vi "Analyze.vi"(8 "error in (no error)":errorcluster, 10 "Image in":T1, 11 "Analyze Total Counts in":refnum<class "Analyze Total Counts.lvclass">) -> (0 "error out":errorcluster, 1 "Result":refnum<class "Analyze Results Base.lvclass">, 2 "Image out":T1, 3 "Analyze Total Counts out":refnum<class "Analyze Total Counts.lvclass">)   [LabVIEW 2020, in "Analyze.lvlib" / "Analyze Total Counts.lvclass"]
uses:
  Analyze Total Counts.lvclass
  C:/POLARIS Programme/POLARIS-AS-3-Cams/Submodules/HIJ Vision/Analyze/Analyze Classes/Analyze BaseClass/Analyze BaseClass/Analyze BaseClass.lvclass
  <vilib>/vision/Image Controls.llb/IMAQ Image.ctl
  Results and Overlays/Results Base/Analyze Results Base.lvclass
  Results and Overlays/Results Total Counts/Analyze Results Total Counts.lvclass
  C:/POLARIS Programme/POLARIS-AS-3-Cams/Submodules/HIJ Vision/Analyze/Results and Overlays/Results Base/Analyze Results Base.lvclass
  Results and Overlays/Results Total Counts/Analyze Results Total Counts.lvclass/Analyze Results Total Counts.ctl
  Results and Overlays/Results Total Counts/Write Total Counts.vi
  Analyze BaseClass/Analyze BaseClass/Analyze BaseClass.lvclass
  <vilib>/vision/NI_Vision_Development_Module.lvlib
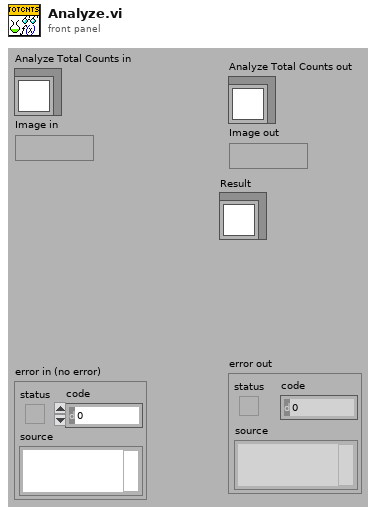
[diagram p1: front panel]
types:
  T1 = typedef "IMAQ Image.ctl" = refnum<image>
  T2 = typedef "ROI Descriptor" = cluster{"Global Rectangle":i32[], "Contours":cluster{"ID":enum32{"External", "Internal"}, "Type":u32, "Coordinates":i32[]}[]}
  T3 = cluster{"Mean Value":sgl, "Standard Variation":sgl, "Minimal Value":sgl, "Maximal Value":sgl, "Area (calibrated)":sgl, "Area (pixels)":u32, "%":sgl, "Calibration Valid":bool}
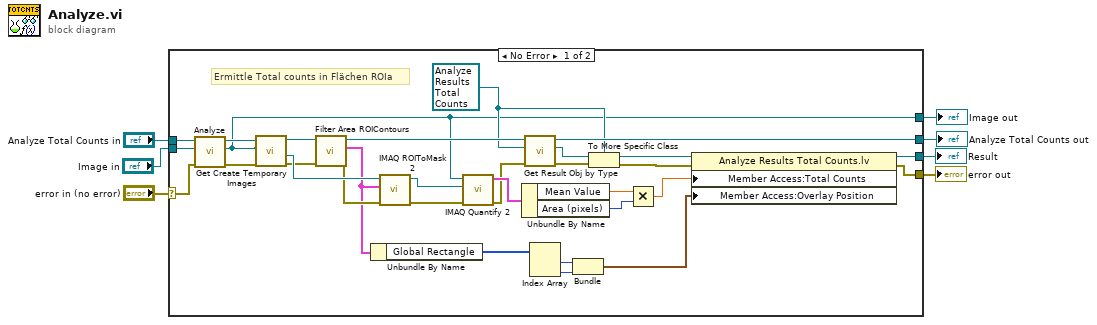
[diagram p0: block diagram]
diagram:
  n1 = case shown="No Error" "error in (no error)" {
    selector: "error in (no error)" -> [w9 w41]
    tunnel: "Image in" -> [w38 w40]
    tunnel: "Analyze Total Counts in" -> [w37 w39]
    tunnel: [w8 w40] -> w5
    tunnel: [w22 w39] -> w4
    tunnel: [w18 _] -> w3
    tunnel: [w15 w41] -> w2
    frame No Error {
      w21 = refnum<class "Analyze Results Total Counts.lvclass"> refnum ("Analyze Results Total Counts.lvclass")
      # "Ermittle Total counts in Flächen ROIa"
      n2 = call-parent "Analyze.vi"("error in (no error)"=w9, "Image in"=w38, "Analyze BaseClass in"=w37) -> ("error out"=w31:errorcluster, "Image out"=w8:T1, "Analyze BaseClass out"=w36:refnum<class "Analyze Total Counts.lvclass">)  [unwired: 5 in, 1 out]
      n3 = call-dynamic "Get Create Temporary Images.vi"("error in (no error)"=w31, "Image in"=w8, "Analyze BaseClass in"=w36) -> ("error out"=w32:errorcluster, "image mask"=w34:T1, "Analyze BaseClass out"=w35:refnum<class "Analyze Total Counts.lvclass">)  [unwired: 4 in, 2 out]
      n4 = call-dynamic "Filter Area ROIContours.vi"("error in (no error)"=w32, "Analyze BaseClass in"=w35) -> ("error out"=w33:errorcluster, "ROI of Area type"=w14:T2, "Analyze BaseClass out"=w23:refnum<class "Analyze Total Counts.lvclass">)  [unwired: 7 in]
      n5 = Unbundle By Name(w14) -> ("Global Rectangle"=w13:i32[])
      n6 = call "IMAQ ROIToMask 2"("error in (no error)"=w33, "ROI Descriptor"=w14, "Image"=w34) -> ("error out"=w29:errorcluster, "Image Out"=w30:T1)  [unwired: 6 in, 1 out]
      n7 = call "IMAQ Quantify 2"("error in (no error)"=w29, "Image Mask"=w30, "Image"=w8) -> ("error out"=w17:errorcluster, "Global Report"=w28:T3)  [unwired: 6 in, 1 out]
      n8 = Unbundle By Name(w28) -> ("Mean Value"=w27:sgl, "Area (pixels)"=w26:u32)
      n9 = call "Get Result Obj by Type.vi"("error in (no error)"=w17, "Parameter Type"=w21, "Analyze BaseClass in"=w23) -> ("error out"=w24:errorcluster, "Parameter"=w25:refnum<class "Analyze Results Base.lvclass">, "Analyze BaseClass out"=w22:refnum<class "Analyze Total Counts.lvclass">)  [unwired: 5 in, 1 out]
      n10 = Index Array(array=w13) -> (element #1=w11:i32, element #2=w12:i32)  [unwired: 2 in]
      n11 = Bundle(w11, w12) -> (w10:cluster{i32, i32})  [unwired: 1 in]
      n12 = To More Specific Class(target class=w21, reference=w25, error in=w24) -> (specific class reference=w20:refnum<class "Analyze Results Total Counts.lvclass">, error out=w16:errorcluster)
      n13 = Multiply(x=w27, y=w26) -> (x*y=w19:sgl)
      n14 = property class="Analyze Results Total Counts.lv"(reference=w20, error in=w16, "Member Access:Total Counts"=w19, "Member Access:Overlay Position"=w10) -> (reference out=w18:refnum<class "Analyze Results Total Counts.lvclass">, error out=w15:errorcluster)
    }
    frame Error {
    }
  }
  "error out" <- w2
  "Analyze Total Counts out" <- w4
  "Image out" <- w5
  "Result" <- w3
